vi "Controls[].vi"(4 "error in (no error)":errorcluster, 6 "Container State":T6, 7 "Display State In":T1={"Item_Refnums_Array"=[], "Root Command"={"Operation"=enum."Add Item", "Data"=variant}}) -> (0 "error out":errorcluster, 2 "Value":refnum<vi>[](array[refnum]), 3 "Display State Out":T1={"Item_Refnums_Array"=[], "Root Command"={"Operation"=enum."Add Item", "Data"=variant}})   [LabVIEW 2011, in "Root_XControl.xctl"]
uses:
  Root_XControl.xctl
  <vilib>/_xctls/Container State.ctl
  State 1.ctl
  Controls/References/Item_Refnums.ctl
  Controls/References/Item_Command_Refnum.ctl
  Controls/Item_Command_Enum.ctl
  Controls/Root_Command.ctl
  Controls/Root_Command_Enum.ctl
  <vilib>/_xctls/XControlSupport.lvlib
panel:
  # "Replace the Value Indicator below with an Indicator of desired type.\nDo not remove this Indicator or the others from the connector pane. \nDo not change the connector pane pattern.\nThe Value Indicator should always be the second terminal from top on the output side in the connector pane."
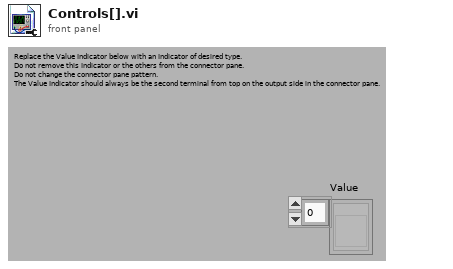
[diagram p1: front panel]
types:
  T1 = typedef "Root_XControl.xctl/State 1.ctl" = cluster{"Item_Refnums_Array":T2[], "Root Command":T4}
  T2 = typedef "Item_Refnums.ctl" = cluster{"VI Refnum":refnum<vi>, "Item_Command_Refnum":T3, "Slide Refnum":refnum<vi>}
  T3 = typedef "Item_Command_Refnum.ctl" = refnum<vi>
  T4 = typedef "Root_Command.ctl" = cluster{"Operation":T5, "Data":variant}
  T5 = typedef "Root_Command_Enum.ctl" = enum16{"Idle", "Add Item", "Delete Item", "Delete All"}
  T6 = typedef "XControlSupport.lvlib/Container State.ctl" = cluster{"Indicator?":bool, "Run Mode?":bool, " Refnum":refnum<vi>}
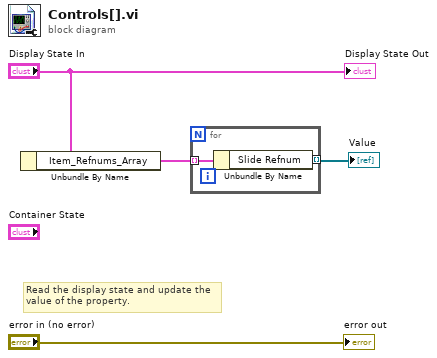
[diagram p0: block diagram]
diagram:
  # "Read the display state and update the value of the property."
  n1 = Unbundle By Name("Display State In") -> ("Item_Refnums_Array"=w2:T2[])
  n2 = for {
    tunnel: w2 -> [w6] mode=indexing
    tunnel: [w5] -> w1 mode=indexing
    n3 = Unbundle By Name(w6) -> ("Slide Refnum"=w5:refnum<vi>)
  }
  "Value" <- w1
  "error out" <- "error in (no error)"
  "Display State Out" <- "Display State In"
